vi "Configure Gamma Correction.vi"(8 "error in (no error)":errorcluster, 9 "Gamma Table Name (\"DEFAULT\")":string="\"DEFAULT\"", 10 "Enable Gamma Correction (T: Enable)":bool=TRUE, 11 "VISA resource name":refnum<visa-resource-name>) -> (0 "error out":errorcluster, 3 "VISA resource name out":refnum<visa-resource-name>)   [LabVIEW 2018, in "Agilent U2000 Series.lvlib"]
doc: "Enables or disables the table-based gamma correction and select the gamma table to be used in the table-based gamma correction.\n\nNote: \nNote:\nThis VI has been obsoleted from the driver and is included for compatibility with existing applications. \n New applications should use the new Public VIs Configure Gamma Table and Enable Gamma Table."
uses:
  Agilent U2000 Series.lvlib
panel:
  # "Note:\nThis VI has been obsoleted from the driver and is included for compatibility with existing applications. \n New applications should use the new Public VIs Configure Gamma Table and Enable Gamma Table."
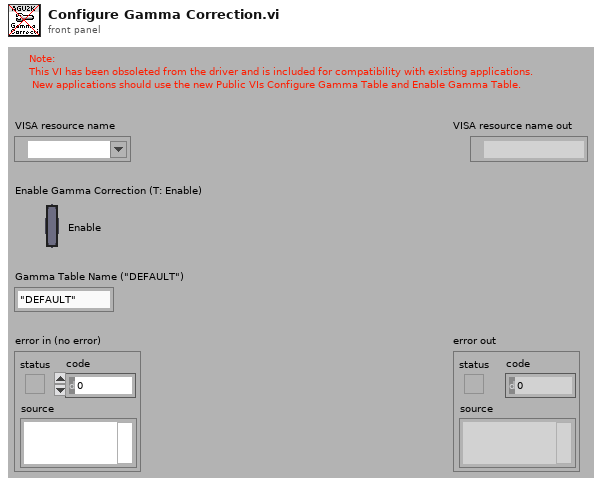
[diagram p1: front panel]
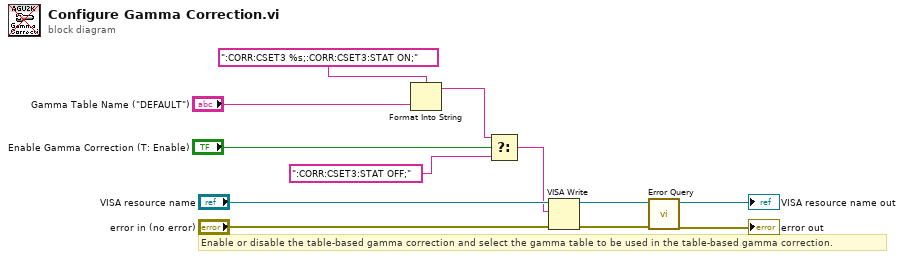
[diagram p0: block diagram]
diagram:
  # "Enable or disable the table-based gamma correction and select the gamma table to be used in the table-based gamma correction."
  n1 = Format Into String(format string=":CORR:CSET3 %s;:CORR:CSET3:STAT ON;", "Gamma Table Name (\"DEFAULT\")") -> (resulting string=w3:string)  [unwired: 2 in, 1 out]
  n2 = Select(t=w3, s="Enable Gamma Correction (T: Enable)", f=":CORR:CSET3:STAT OFF;") -> (s? t:f=w1:string)
  n3 = VISA Write(VISA resource name="VISA resource name", write buffer=w1, error in (no error)="error in (no error)") -> (VISA resource name out=w9:refnum<visa-resource-name>, error out=w8:errorcluster)  [unwired: 1 out]
  n4 = call "Error Query.vi"("error in (no error)"=w8, "VISA resource name"=w9) -> ("error out"=→"error out":errorcluster, "VISA resource name out"=→"VISA resource name out":refnum<visa-resource-name>)  [unwired: 6 in, 2 out]
